vi "Test Hardware ID Import.vi"() -> ()   [LabVIEW 2012]
panel:
  out "cfg hash equal?":bool
  out "hash 3 equal?":bool
  out "hash 2 equal?":bool
  out "hash 1 equal?":bool
  out "Cfg Hash":string[](array[string])
  out "Hash 3":string[](array[string])
  out "Hash 2":string[](array[string])
  out "Hash 1":string[](array[string])
  in  "Lockout Date 3":timestamp format="%<%x>T"
  in  "Lockout Date 1":timestamp format="%<%x>T"
  in  "Lockout Date 2":timestamp format="%<%x>T"
  in  "ID":string
  out "hidOutnoNull":string
  out "hidOut":string
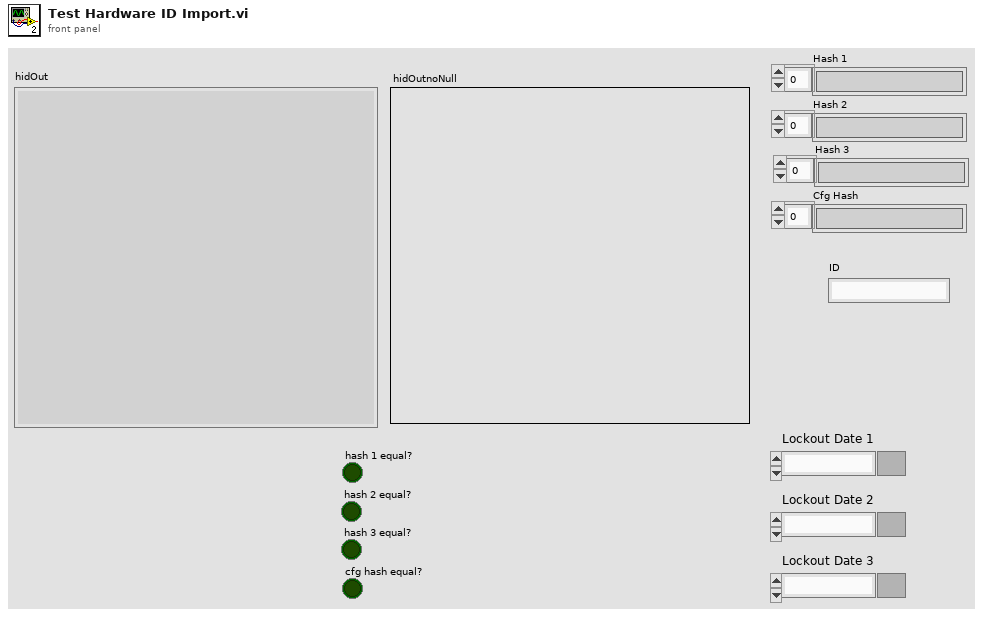
[diagram p1: front panel]
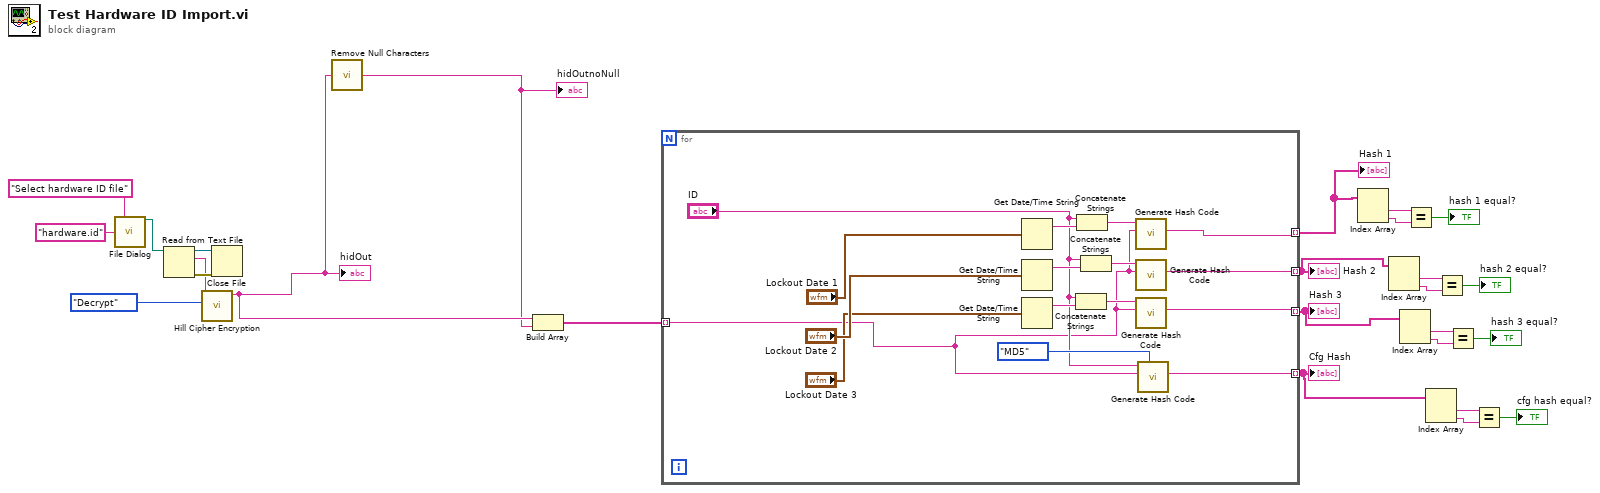
[diagram p0: block diagram]
diagram:
  n1 = call "File Dialog"("prompt"="Select hardware ID file", "default name"="hardware.id") -> ("selected path"=w23:path)  [unwired: 10 in, 3 out]
  n2 = Read from Text File(file (use dialog)=w23) -> (refnum out=w21:refnum<file>, text=w20:string, error out=w22:errorcluster)  [unwired: 3 in, 1 out]
  n3 = call <userlib>:"Hill Cipher Encryption.vi"("Operation"=enum16{"Encrypt", "Decrypt", "Decrypt from Hex"}."Decrypt", "Input String"=w20) -> ("Output String"=w18:string)  [unwired: 7 in, 2 out]
  "hidOut" <- w18
  n4 = Close File(refnum=w21, error in=w22) -> ()  [unwired: 2 out]
  n5 = call "Remove Null Characters.vi"("strIn"=w18) -> ("strOut"=w17:string)  [unwired: 4 in]
  "hidOutnoNull" <- w17
  n6 = Build Array(w18, w17) -> (w19:string[])
  n7 = for {
    tunnel: [w31] -> w16 mode=indexing
    tunnel: [w30] -> w9 mode=indexing
    tunnel: [w29] -> w5 mode=indexing
    tunnel: [w28] -> w1 mode=indexing
    tunnel: w19 -> [w27] mode=indexing
    n8 = Get Date/Time String(seconds (now)="Lockout Date 1") -> (date string=w36:string)  [unwired: 2 in, 1 out]
    n9 = Get Date/Time String(seconds (now)="Lockout Date 2") -> (date string=w37:string)  [unwired: 2 in, 1 out]
    n10 = Get Date/Time String(seconds (now)="Lockout Date 3") -> (date string=w38:string)  [unwired: 2 in, 1 out]
    n11 = Concatenate Strings("ID", w38) -> (w41:string)
    n12 = Concatenate Strings("ID", w36) -> (w39:string)
    n13 = Concatenate Strings("ID", w37) -> (w40:string)
    n14 = call "Generate Hash Code.vi"("Fingerprint"=w27, "Product ID"=w39) -> ("Hash"=w31:string)  [unwired: 8 in, 1 out]
    n15 = call "Generate Hash Code.vi"("Fingerprint"=w27, "Product ID"=w40) -> ("Hash"=w30:string)  [unwired: 8 in, 1 out]
    n16 = call "Generate Hash Code.vi"("Fingerprint"=w27, "Product ID"=w41) -> ("Hash"=w29:string)  [unwired: 8 in, 1 out]
    n17 = call "Generate Hash Code.vi"("Hash"=enum16{"MD5", "FNV-1"}."MD5", "Fingerprint"=w27, "Product ID"="ID") -> ("Hash"=w28:string)  [unwired: 7 in, 1 out]
  }
  "Hash 1" <- w16
  "Hash 2" <- w9
  "Hash 3" <- w5
  "Cfg Hash" <- w1
  n18 = Index Array(array=w16) -> (element #1=w14:string, element #2=w15:string)  [unwired: 2 in]
  n19 = Index Array(array=w9) -> (element #1=w11:string, element #2=w10:string)  [unwired: 2 in]
  n20 = Index Array(array=w5) -> (element #1=w7:string, element #2=w8:string)  [unwired: 2 in]
  n21 = Equal?(x=w14, y=w15) -> (x = y?=→"hash 1 equal?":bool)
  n22 = Index Array(array=w1) -> (element #1=w3:string, element #2=w2:string)  [unwired: 2 in]
  n23 = Equal?(x=w11, y=w10) -> (x = y?=→"hash 2 equal?":bool)
  n24 = Equal?(x=w7, y=w8) -> (x = y?=→"hash 3 equal?":bool)
  n25 = Equal?(x=w3, y=w2) -> (x = y?=→"cfg hash equal?":bool)
